vi "DAQ_measure_QPD_signal.vi"(2 "Reset":bool, 3 "error in":errorcluster, 5 "display options":cluster{"init":bool, "selection":u16}) -> (0 "error out":errorcluster, 1 "Waveform Chart":cluster{"mean":dbl, "mean":dbl, "mean":dbl}(graph))   [LabVIEW 2015]
uses:
  <vilib>/Analysis/NI_AALBase.lvlib
  <vilib>/Analysis/baseanly.llb/Mean (DBL).vi
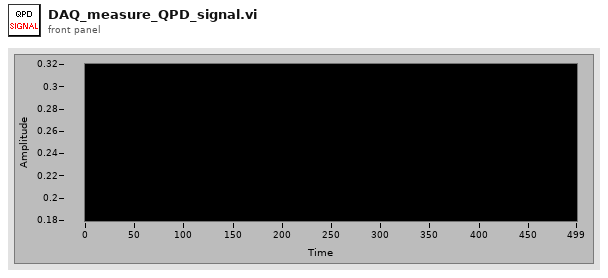
[diagram p1: front panel]
types:
  T1 = enum16{"Always On", "Always Off", "Off While Running"}
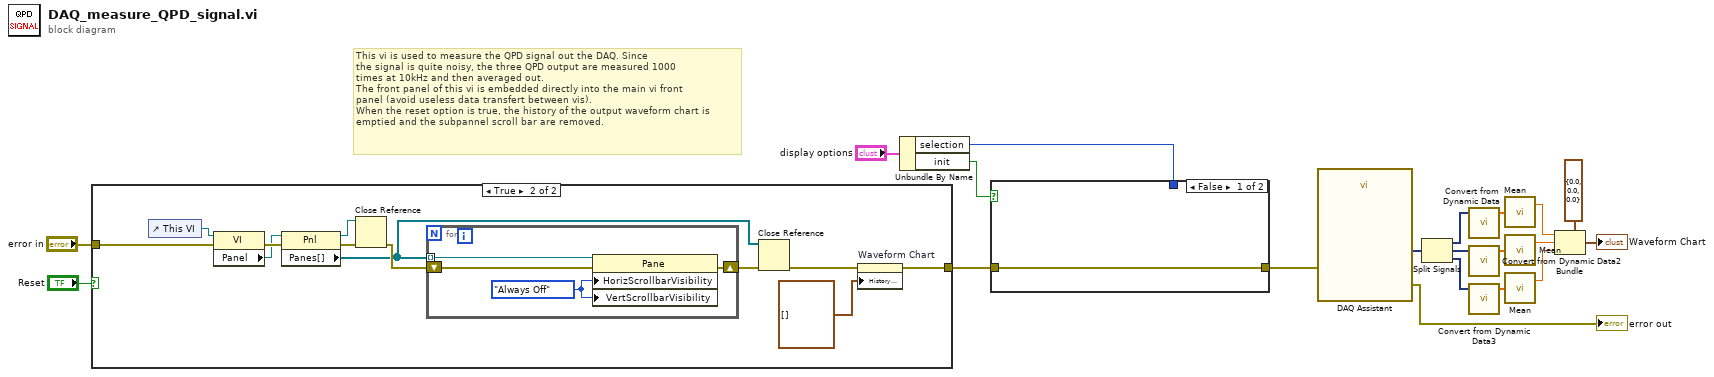
[diagram p0: block diagram]
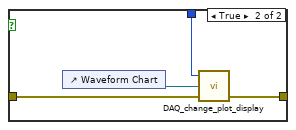
[diagram p2: hidden frame]
diagram:
  # "This vi is used to measure the QPD signal out the DAQ. Since\nthe signal is quite noisy, the three QPD output are measured 1000\ntimes at 10kHz and then averaged out.\nThe front panel of this vi is embedded directly into the main vi front\npanel (avoid useless data transfert between vis). \nWhen the reset option is true, the history of the output waveform chart is\nemptied and the subpannel scroll bar are removed."
  n1 = case shown="True" "Reset" {
    tunnel: "error in" -> [w21 w25]
    tunnel: [w21 w22] -> w4
    frame False {
    }
    frame True {
      n2 = control-ref of="This VI"() -> (w26:refnum<vi>)
      n3 = property class="VI"(reference=w26, error in=w25) -> (error out=w28:errorcluster, "Panel"=w27:refnum<vi>)  [unwired: 1 out]
      n4 = property class="Pnl"(reference=w27, error in=w28) -> (reference out=w29:refnum<vi>, error out=w30:errorcluster, "Panes[]"=w32:refnum<vi>[])
      n5 = Close Reference(reference=w29, error in (no error)=w30) -> (error out=w33:errorcluster)
      n6 = for {
        tunnel: w32 -> [w37] mode=indexing
        shift-right: [w35] -> w31
        shift-left: w33 -> [w34]
        w36 = T1."Always Off" ("Horizontal Scrollbar Visibility")
        n7 = property class="Pane"(reference=w37, error in=w34, "HorizScrollbarVisibility"=w36, "VertScrollbarVisibility"=w36) -> (error out=w35:errorcluster)  [unwired: 1 out]
      }
      n8 = Close Reference(reference=w32, error in (no error)=w31) -> (error out=w24:errorcluster)
      n9 = property on="Waveform Chart" class="WFChart (strict)"(error in=w24, "History Data"=cluster{"mean":dbl, "mean":dbl, "mean":dbl}[] []) -> (error out=w22:errorcluster)  [unwired: 1 in, 1 out]
    }
  }
  n10 = Unbundle By Name("display options") -> ("selection"=w3:u16, "init"=w5:bool)
  n11 = case shown="False" w5 {
    tunnel: w4 -> [w38 w42]
    tunnel: [w38 w41] -> w2
    tunnel: w3 -> [_ w39]
    frame False {
    }
    frame True {
      n12 = control-ref of="Waveform Chart"() -> (w40:refnum<vi>)
      n13 = call "DAQ_change_plot_display.vi"("error in"=w42, "WFChart Refnum"=w40, "selection"=w39) -> ("error out"=w41:errorcluster)  [unwired: 2 in]
    }
  }
  n14 = call "DAQ Assistant"("error in"=w2) -> ("data"=w9:dynamicdata, "error out"=→"error out":errorcluster)  [unwired: 16 in, 1 out]
  n15 = Split Signals(w9) -> (w20:dynamicdata, w16:dynamicdata, w15:dynamicdata)  [unwired: 3 in]
  n16 = call "Convert from Dynamic Data"("Dynamic Data Type"=w20) -> ("Array"=w19:dbl[])  [unwired: 3 in]
  n17 = call "Convert from Dynamic Data2"("Dynamic Data Type"=w16) -> ("Array"=w18:dbl[])  [unwired: 3 in]
  n18 = call "Convert from Dynamic Data3"("Dynamic Data Type"=w15) -> ("Array"=w17:dbl[])  [unwired: 3 in]
  n19 = call-poly <vilib>:"Mean.vi"("X"=w19) -> ("mean"=w14:dbl)  [unwired: 1 out]
  n20 = call-poly <vilib>:"Mean.vi"("X"=w18) -> ("mean"=w13:dbl)  [unwired: 1 out]
  n21 = call-poly <vilib>:"Mean.vi"("X"=w17) -> ("mean"=w12:dbl)  [unwired: 1 out]
  n22 = Bundle(cluster=cluster{"mean":dbl, "mean":dbl, "mean":dbl} {"mean"=0.0, "mean"=0.0, "mean"=0.0} ("output cluster"), "mean"=w14, "mean"=w13, "mean"=w12) -> (→"Waveform Chart":cluster{"mean":dbl, "mean":dbl, "mean":dbl})
